vi "Read Format string.vi"(8 "error in (no error)":errorcluster, 11 "Floating point base in":refnum<class "Floating point base.lvclass">) -> (0 "error out":errorcluster, 2 "Format string":string, 3 "Floating point base out":refnum<class "Floating point base.lvclass">)   [LabVIEW 2018, in "D Datagrid Library.lvlib" / "Floating point base.lvclass"]
uses:
  Floating point base.lvclass
  Floating point base.lvclass/Floating point base.ctl
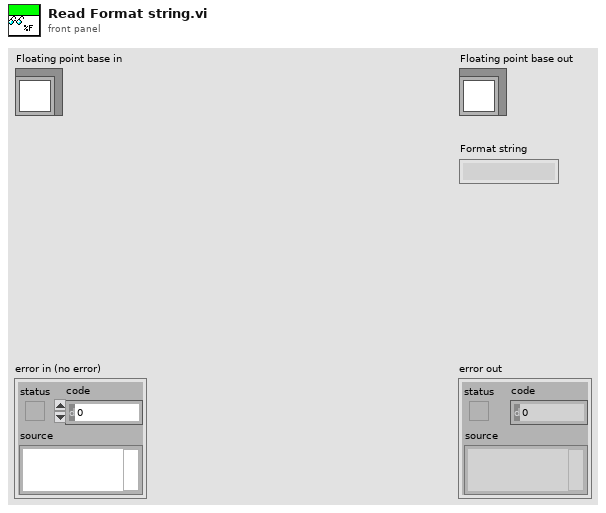
[diagram p1: front panel]
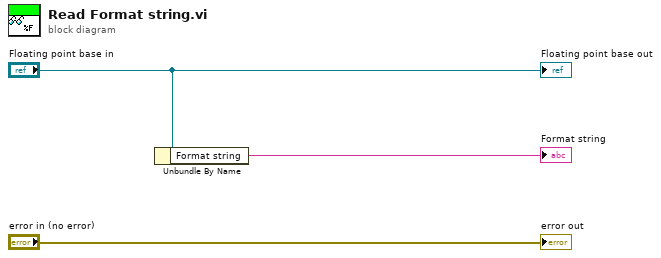
[diagram p0: block diagram]
diagram:
  n1 = Unbundle By Name("Floating point base in") -> ("Format string"=→"Format string":string)
  "error out" <- "error in (no error)"
  "Floating point base out" <- "Floating point base in"
